vi "Configure Trigger Basic.vi"(5 "Trigger Mode (0: Auto)":i32(ring) items=["Auto", "Normal"], 6 "Trigger Type (0: Edge)":i32(ring) items=["Edge", "Pulse", "Slope", "Video", "Runt", "Prunt", "Pattern", "Nth Edge", "Delay", "Timeout", "Setup/Hold"], 8 "error in (no error)":errorcluster, 9 "Holdoff Time (0 s)":dbl, 10 "Coupling Mode (0: AC)":i32(ring) items=["AC", "DC", "LF Reject", "HF Reject"], 11 "VISA resource name":refnum<visa-resource-name>) -> (0 "error out":errorcluster, 3 "VISA resource name out":refnum<visa-resource-name>)   [LabVIEW 2015, in "ZhiYuan ZDS Series for TCP.lvlib"]
doc: "Configures the basic setting for trigger."
uses:
  ZhiYuan ZDS Series for TCP.lvlib
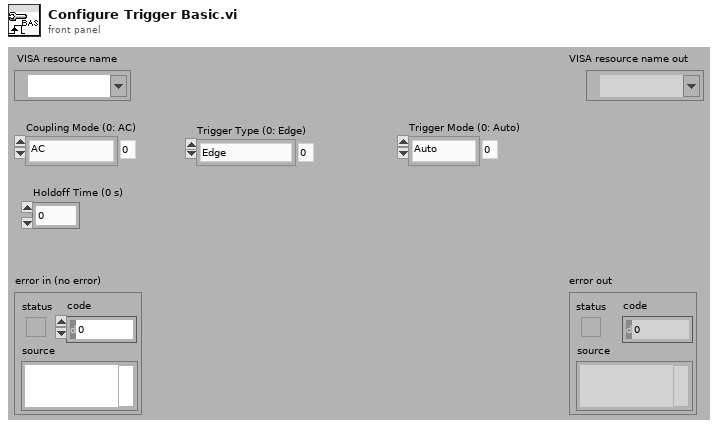
[diagram p1: front panel]
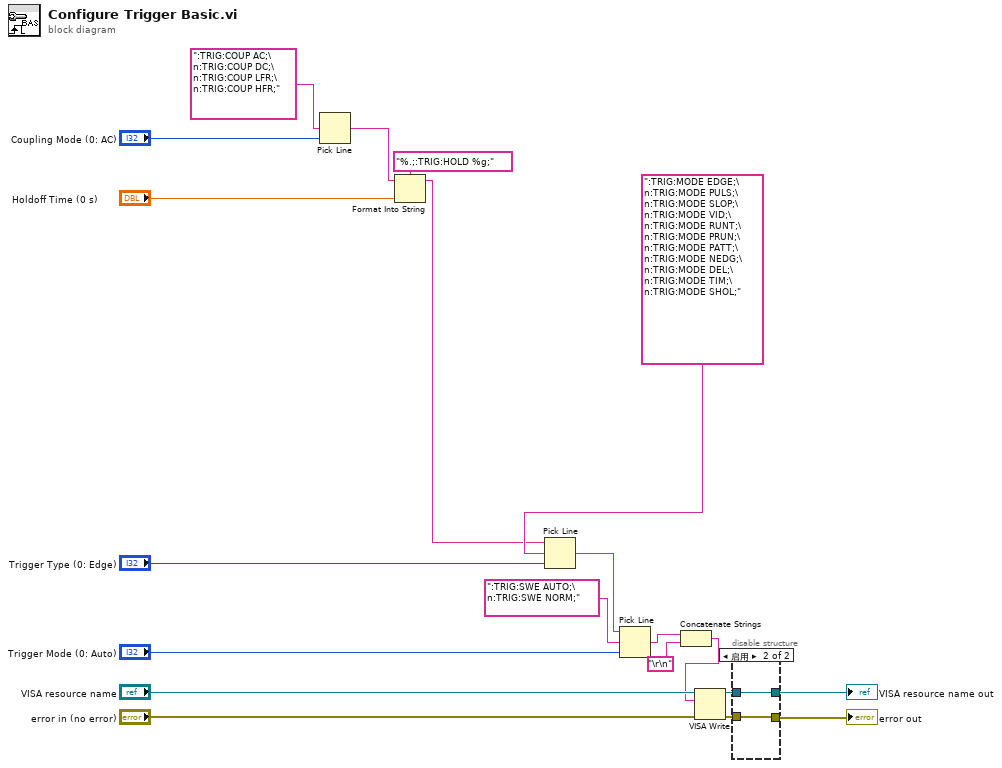
[diagram p0: block diagram]
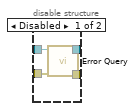
[diagram p2: hidden frame]
diagram:
  n1 = Pick Line(multi-line string=":TRIG:COUP AC;\n:TRIG:COUP DC;\n:TRIG:COUP LFR;\n:TRIG:COUP HFR;", line index="Coupling Mode (0: AC)") -> (output string=w18:string)  [unwired: 1 in]
  n2 = Format Into String(format string="%.;:TRIG:HOLD %g;", initial string=w18, "Holdoff Time (0 s)") -> (resulting string=w4:string)  [unwired: 1 in, 1 out]
  n3 = Pick Line(string ("")=w4, multi-line string=":TRIG:MODE EDGE;\n:TRIG:MODE PULS;\n:TRIG:MODE SLOP;\n:TRIG:MODE VID;\n:TRIG:MODE RUNT;\n:TRIG:MODE PRUN;\n:TRIG:MODE PATT;\n:TRIG:MODE NEDG;\n:TRIG:MODE DEL;\n:TRIG:MODE TIM;\n:TRIG:MODE SHOL;", line index="Trigger Type (0: Edge)") -> (output string=w11:string)
  n4 = Pick Line(string ("")=w11, multi-line string=":TRIG:SWE AUTO;\n:TRIG:SWE NORM;", line index="Trigger Mode (0: Auto)") -> (output string=w3:string)
  n5 = Concatenate Strings(w3, "\r\n") -> (w1:string)
  n6 = VISA Write(VISA resource name="VISA resource name", write buffer=w1, error in (no error)="error in (no error)") -> (VISA resource name out=w8:refnum<visa-resource-name>, error out=w7:errorcluster)  [unwired: 1 out]
  n7 = disable-structure shown="启用" {
    disable-tunnel: w8 -> [w24 w25]
    disable-tunnel: w7 -> [w23 w26]
    disable-tunnel: [w22 w25] -> w6
    disable-tunnel: [w21 w26] -> w5
    frame Disabled {
      n8 = call "Error Query.vi"("error in (no error)"=w23, "VISA resource name"=w24) -> ("error out"=w21:errorcluster, "VISA resource name out"=w22:refnum<visa-resource-name>)  [unwired: 6 in, 2 out]
    }
    frame Enabled {
    }
  }
  "VISA resource name out" <- w6
  "error out" <- w5
